vi "swap.vi"(4 "j":i32, 6 "k":u32, 11 "Array":dbl[](array[numeric])) -> (3 "Array (swap)":dbl[](array[numeric]))   [LabVIEW 2014]
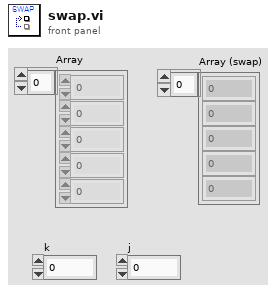
[diagram p1: front panel]
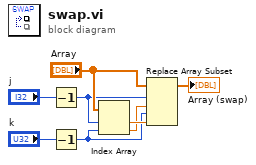
[diagram p0: block diagram]
diagram:
  n1 = Decrement(x="j") -> (x-1=w2:i32)
  n2 = Decrement(x="k") -> (x-1=w1:u32)
  n3 = Index Array(array="Array", index #1=w2, index #2=w1) -> (element #1=w7:dbl, element #2=w5:dbl)
  n4 = Replace Array Subset(array="Array", new element #1=w5, index #1=w2, new element #2=w7, index #2=w1) -> (→"Array (swap)":dbl[])
